vi "CSDB_Config.write 2 DB.vi"(1 "ClassName":string, 2 "AttributeNames":string[](array[string]), 3 "Values":string[][](array[string]), 4 "InstanceNames":string[](array[string]), 5 "error in (no error)":errorcluster, 10 "new instances?":bool) -> (19 "error out":errorcluster)   [LabVIEW 2014, in "CSDB_Config.lvlib"]
doc: "Writes values to the database"
uses:
  CSDB_Config.lvlib
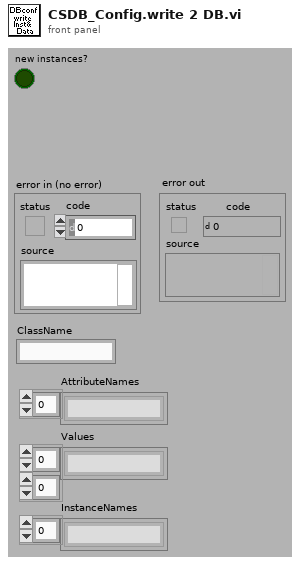
[diagram p1: front panel]
types:
  T1 = enum16{"Left Button", "Center Button", "Right Button", "Window Close"}
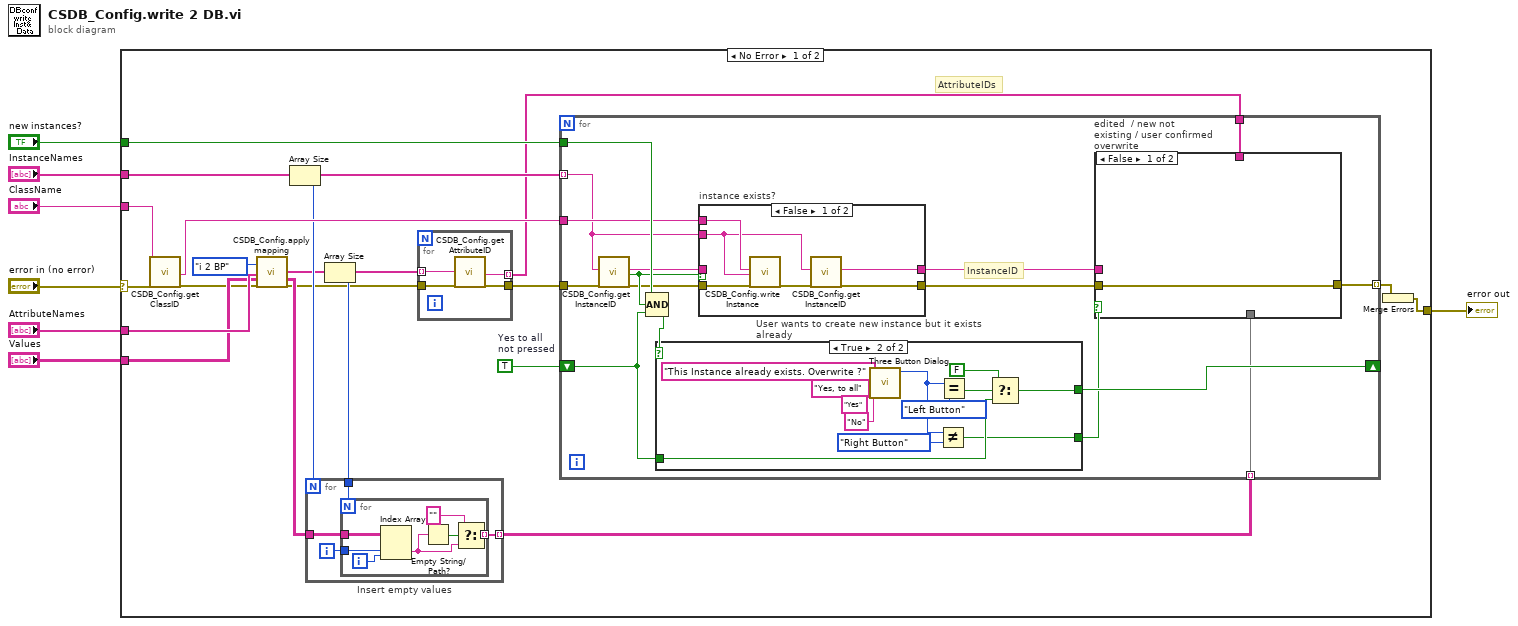
[diagram p0: block diagram]
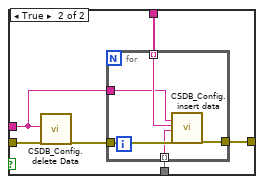
[diagram p3: hidden frame]
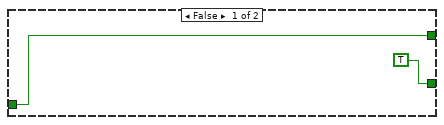
[diagram p4: hidden frame]
diagram:
  n1 = case shown="No Error" "error in (no error)" {
    selector: "error in (no error)" -> [w8 w93]
    tunnel: "AttributeNames" -> [w27 _]
    tunnel: "Values" -> [w25 _]
    tunnel: "ClassName" -> [w24 _]
    tunnel: "new instances?" -> [w22 _]
    tunnel: "InstanceNames" -> [w19 _]
    tunnel: [w9 w93] -> w2
    frame No Error {
      w21 = TRUE  # Yes to all not pressed
      # "AttributeIDs"
      n2 = call "CSDB_Config.get ClassID.vi"("ClassName"=w24, "error in (no error)"=w8) -> ("ClassID"=w20:string, "error out"=w23:errorcluster)  [unwired: 16 in]
      n3 = call "CSDB_Config.apply mapping.vi"("Enum"=enum16{"i 2 BP", "BP 2 i", "get"}."i 2 BP", "AttributeNamesIn"=w27, "Values in"=w25, "error in (no error)"=w23) -> ("AttributeNames out"=w13:string[], "Values out"=w16:string[][], "error out"=w15:errorcluster)  [unwired: 13 in]
      n4 = Array Size(array=w19) -> (size(s)=w18:i32)
      n5 = Array Size(array=w13) -> (size(s)=w17:i32)
      n6 = for "Insert empty values" {
        N: w18 -> [_]
        tunnel: [w32] -> w11 mode=indexing
        tunnel: w16 -> [w35]
        tunnel: w17 -> [w34]
        i -> [w33]
        n7 = for {
          N: w34 -> [_]
          tunnel: w35 -> [w42]
          tunnel: w33 -> [w41]
          tunnel: [w36] -> w32 mode=indexing
          i -> [w40]
          n8 = Index Array(array=w42, index (row)=w41, index (col)=w40) -> (element=w38:string)
          n9 = Empty String/Path?(string/path=w38) -> (empty?=w39:bool)
          n10 = Select(t="", s=w39, f=w38) -> (s? t:f=w36:string)
        }
      }
      n11 = for {
        tunnel: w15 -> [w31]
        tunnel: [w30] -> w14
        tunnel: w13 -> [w29] mode=indexing
        tunnel: [w28] -> w12 mode=indexing
        n12 = call "CSDB_Config.get AttributeID.vi"("AttributeName"=w29, "error in (no error)"=w31) -> ("AttributeID"=w28:string, "error out"=w30:errorcluster)  [unwired: 16 in]
      }
      n13 = for {
        tunnel: w14 -> [w58]
        tunnel: w19 -> [w49] mode=indexing
        tunnel: w22 -> [w57]
        shift-right: [w54] -> _
        shift-left: w21 -> [w55]
        tunnel: w20 -> [w50]
        tunnel: w12 -> [w47]
        tunnel: w11 -> [w44] mode=indexing
        tunnel: [w43] -> w10 mode=indexing
        # "InstanceID"
        n14 = call "CSDB_Config.get InstanceID.vi"("InstanceName"=w49, "error in (no error)"=w58) -> ("InstanceID"=w45:string, "entry exists?"=w52:bool, "error out"=w51:errorcluster)  [unwired: 15 in]
        n15 = Compound Arithmetic op=AND(w57, w52, w55) -> (w56:bool)
        n16 = case "User wants to create new instance but it exists already" shown="True" w56 {
          tunnel: w55 -> [w80 w86]
          tunnel: [w80 w84] -> w54
          tunnel: [TRUE w81] -> w53
          frame False {
          }
          frame True {
            n17 = call <vilib>:"Three Button Dialog.vi"("Right Button Text (\"Cancel\")"="No" ("Right Button Text (\"Cancel\")"), "Center Button Text (\"No\")"="Yes" ("Center Button Text (\"No\")"), "Left Button Text (\"Yes\")"="Yes, to all" ("Left Button Text (\"Yes\")"), "message"="This Instance already exists. Overwrite ?") -> ("Which Button?"=w83:T1)  [unwired: 7 in]
            n18 = Not Equal?(x=w83, y=T1."Right Button") -> (x != y?=w81:bool)
            n19 = Equal?(x=w83, y=T1."Left Button") -> (x = y?=w87:bool)
            n20 = Select(t=FALSE, s=w87, f=w86) -> (s? t:f=w84:bool)
          }
        }
        n21 = case "instance exists?" shown="False" w52 {
          tunnel: w51 -> [w64 w66]
          tunnel: w50 -> [w63 _]
          tunnel: w49 -> [w60 _]
          tunnel: [w61 w66] -> w48
          tunnel: [w59 w65] -> w46
          tunnel: w45 -> [_ w65]
          frame False {
            n22 = call "CSDB_Config.write Instance.vi"("ClassID"=w63, "InstanceName"=w60, "error in (no error)"=w64) -> ("error out"=w62:errorcluster)  [unwired: 16 in]
            n23 = call "CSDB_Config.get InstanceID.vi"("InstanceName"=w60, "error in (no error)"=w62) -> ("InstanceID"=w59:string, "error out"=w61:errorcluster)  [unwired: 15 in, 1 out]
          }
          frame True {
          }
        }
        n24 = case "edited  / new not existing / user confirmed overwrite" shown="False" w53 {
          tunnel: w48 -> [w67 w73]
          tunnel: w47 -> [_ w71]
          tunnel: w46 -> [_ w70]
          tunnel: w44 -> [_ w69]
          tunnel: [w67 w68] -> w43
          frame False {
          }
          frame True {
            n25 = call "CSDB_Config.delete Data.vi"("InstanceID"=w70, "error in (no error)"=w73) -> ("error out"=w72:errorcluster)  [unwired: 17 in]
            n26 = for {
              tunnel: w72 -> [w78]
              tunnel: w71 -> [w77] mode=indexing
              tunnel: w70 -> [w76]
              tunnel: w69 -> [w75] mode=indexing
              tunnel: [w74] -> w68
              n27 = call "CSDB_Config.insert data.vi"("InstanceID"=w76, "AttributeID"=w77, "Value"=w75, "error in (no error)"=w78) -> ("error out"=w74:errorcluster)  [unwired: 15 in]
            }
          }
        }
      }
      n28 = Merge Errors(w10) -> (w9:errorcluster)
    }
    frame Error {
    }
  }
  "error out" <- w2
